vi "weightedAccumulator.vi"(7 "reset":bool, 10 "weight":fxp<+,16,0>, 11 "input":i16) -> (3 "weightedSum":fxp<+/-,54,34>)   [LabVIEW 2016]
uses:
  <vilib>/rvi/FXPMathLib/FxpAdd/XNode/nifxpmath_Add.xnode
  <vilib>/rvi/FXPMathLib/FxpInterpret/XNode/nifxpmath_Interpret.xnode
  <vilib>/rvi/FXPMathLib/FxpMul/XNode/nifxpmath_Multiplier.xnode
  <vilib>/rvi/FXPMathLib/sim/FxpSim.dll
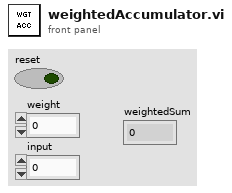
[diagram p1: front panel]
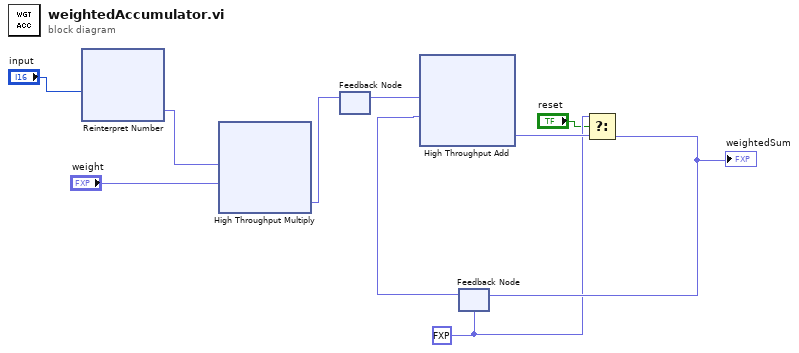
[diagram p0: block diagram]
diagram:
  w3 = fxp<+/-,53,33> 0.0 ("x+y")
  n1 = xnode "Reinterpret Number"("x"="input") -> ("y"=w6:fxp<+/-,16,16>)
  n2 = xnode ("High Throughput Multiply")("x"=w6, "y"="weight") -> ("x*y"=w8:fxp<+/-,32,16>)
  n3 = feedback-in #1(w8) -> ()
  n4 = feedback #1() -> (w1:fxp<+/-,32,16>)  [unwired: 1 in]
  n5 = feedback #2(w3) -> (w5:fxp<+/-,53,33>)
  n6 = xnode ("High Throughput Add")("x"=w1, "y"=w5) -> ("x+y"=w9:fxp<+/-,52,32>)
  n7 = Select(t=w3, s="reset", f=w9) -> (s? t:f=w4:fxp<+/-,53,33>)
  "weightedSum" <- w4
  n8 = feedback-in #2(w4) -> ()
